vi "Move_Block_Down.vi"(10 "old Block":T1 {"orientaion" items=["up", "down", "left", "right"]; "type" items=["t", "rl", "ll", "rz", "lz", "square", "line"]}) -> (2 "new Block":T1 {"orientaion" items=["up", "down", "left", "right"]; "type" items=["t", "rl", "ll", "rz", "lz", "square", "line"]})   [LabVIEW 2015]
uses:
  block.ctl
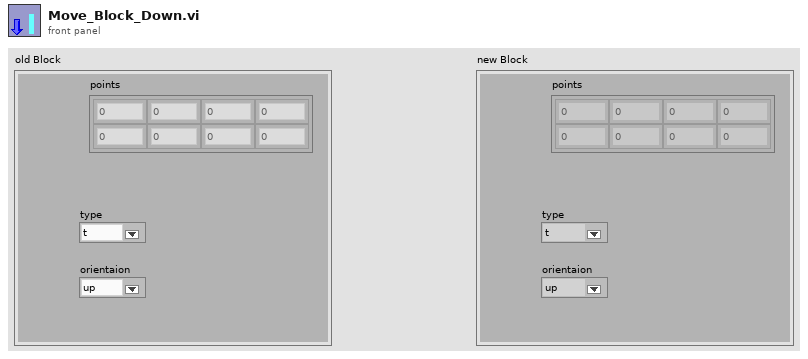
[diagram p1: front panel]
types:
  T1 = typedef "block.ctl" = cluster{"points":dbl[][], "type":u16, "orientaion":u16}
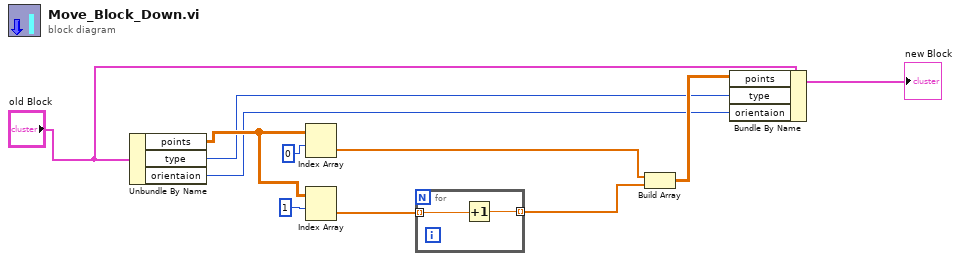
[diagram p0: block diagram]
diagram:
  n1 = Unbundle By Name("old Block") -> ("points"=w9:dbl[][], "type"=w2:u16, "orientaion"=w1:u16)
  n2 = Index Array(array=w9, index (row)=0) -> (element=w7:dbl[])  [unwired: 1 in]
  n3 = Index Array(array=w9, index (row)=1) -> (element=w8:dbl[])  [unwired: 1 in]
  n4 = for {
    tunnel: w8 -> [w13] mode=indexing
    tunnel: [w12] -> w6 mode=indexing
    n5 = Increment(x=w13) -> (x+1=w12:dbl)
  }
  n6 = Build Array(w7, w6) -> (w5:dbl[][])
  n7 = Bundle By Name(cluster="old Block", "points"=w5, "type"=w2, "orientaion"=w1) -> (→"new Block":T1)
